vi "dequeue.vi"(8 "error in (no error)":errorcluster, 11 "ComicVine_manager in":refnum<class "CV_downloader.lvclass">) -> (0 "error out":errorcluster, 1 "data":variant, 2 "cmd":T1, 3 "ComicVine_manager out":refnum<class "CV_downloader.lvclass">)   [LabVIEW 2024, in "CV_downloader.lvclass"]
uses:
  CV_downloader.lvclass
  states--enum.ctl
  CV_downloader.lvclass/CV_downloader.ctl
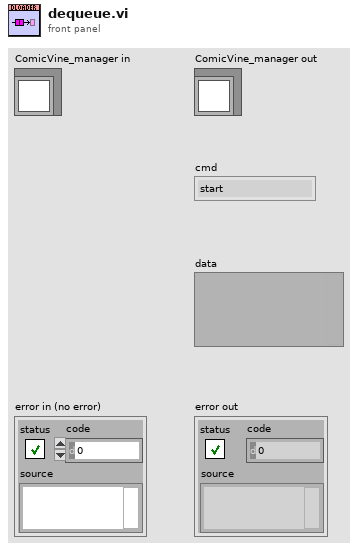
[diagram p1: front panel]
types:
  T1 = typedef "CV_downloader.lvclass/states--enum.ctl" = enum16{"start", "running", "start timer", "update file", "set directories", "wait", "shutdown"}
  T2 = typedef "CV_downloader.lvclass/queue.message--cluster.ctl" = cluster{"cmd":T1, "data":variant}
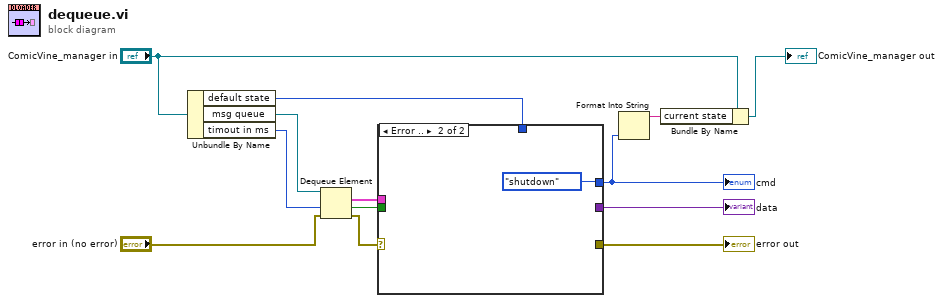
[diagram p0: block diagram]
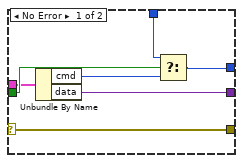
[diagram p2: hidden frame]
diagram:
  n1 = Unbundle By Name("ComicVine_manager in") -> ("default state"=w9:T1, "msg queue"=w12:refnum<queue>, "timout in ms"=w13:i32)
  n2 = Dequeue Element(queue=w12, timeout in ms (-1)=w13, error in (no error)="error in (no error)") -> (element=w10:T2, timed out?=w11:bool, error out=w6:errorcluster)  [unwired: 1 out]
  n3 = case shown="Error .." w6 {
    selector: w6 -> [w14 _]
    tunnel: w11 -> [w20 _]
    tunnel: w10 -> [w19 _]
    tunnel: w9 -> [w17 _]
    tunnel: [w16 _] -> w7
    tunnel: [w15 states--enum."shutdown" ("cmd")] -> w4
    tunnel: [w14 _] -> w5
    frame No Error {
      n4 = Unbundle By Name(w19) -> ("cmd"=w18:T1, "data"=w16:variant)
      n5 = Select(t=w17, s=w20, f=w18) -> (s? t:f=w15:T1)
    }
    frame Error {
    }
  }
  "error out" <- w5
  "data" <- w7
  "cmd" <- w4
  n6 = Format Into String(w4) -> (resulting string=w3:string)  [unwired: 3 in, 1 out]
  n7 = Bundle By Name(cluster="ComicVine_manager in", "current state"=w3) -> (→"ComicVine_manager out":refnum<class "CV_downloader.lvclass">)
